vi "Save Analyzed Booth.vi"(8 "Error In":errorcluster, 10 "File Path":path, 11 "Data cluster":T1) -> (0 "Error Out":errorcluster)   [LabVIEW 2019, in "SubVIs.lvlib"]
uses:
  SubVIs.lvlib
  Controls/Save Data Cluster.ctl
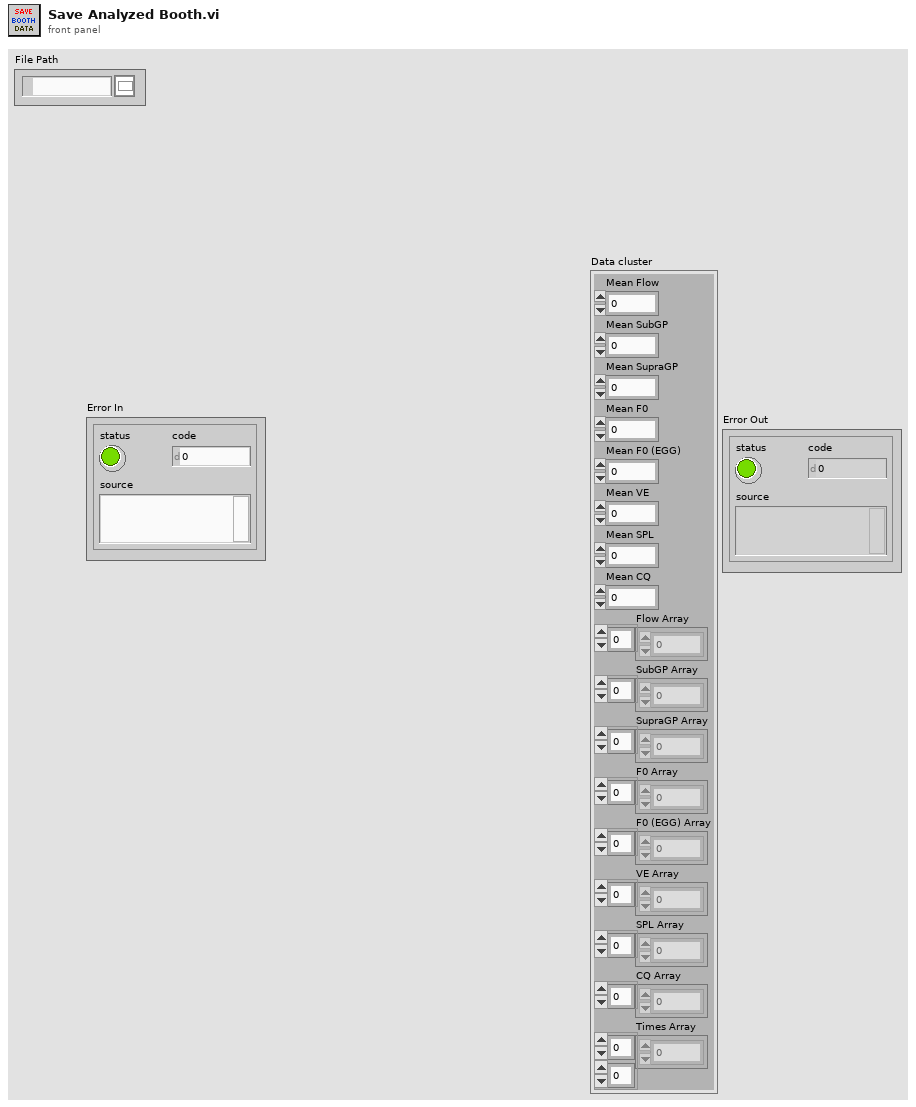
[diagram p1: front panel]
types:
  T1 = typedef "Save Data Cluster.ctl" = cluster{"Mean Flow":dbl, "Mean SubGP":dbl, "Mean SupraGP":dbl, "Mean F0":dbl, "Mean F0 (EGG)":dbl, "Mean VE":dbl, "Mean SPL":dbl, "Mean CQ":dbl, "Flow Array":dbl[], "SubGP Array":dbl[], "SupraGP Array":dbl[], "F0 Array":dbl[], "F0 (EGG) Array":dbl[], "VE Array":dbl[], "SPL Array":dbl[], "CQ Array":dbl[], "Times Array":dbl[][]}
  T2 = enum16{"open", "replace", "create", "open or create", "replace or create", "replace or create with confirmation"}
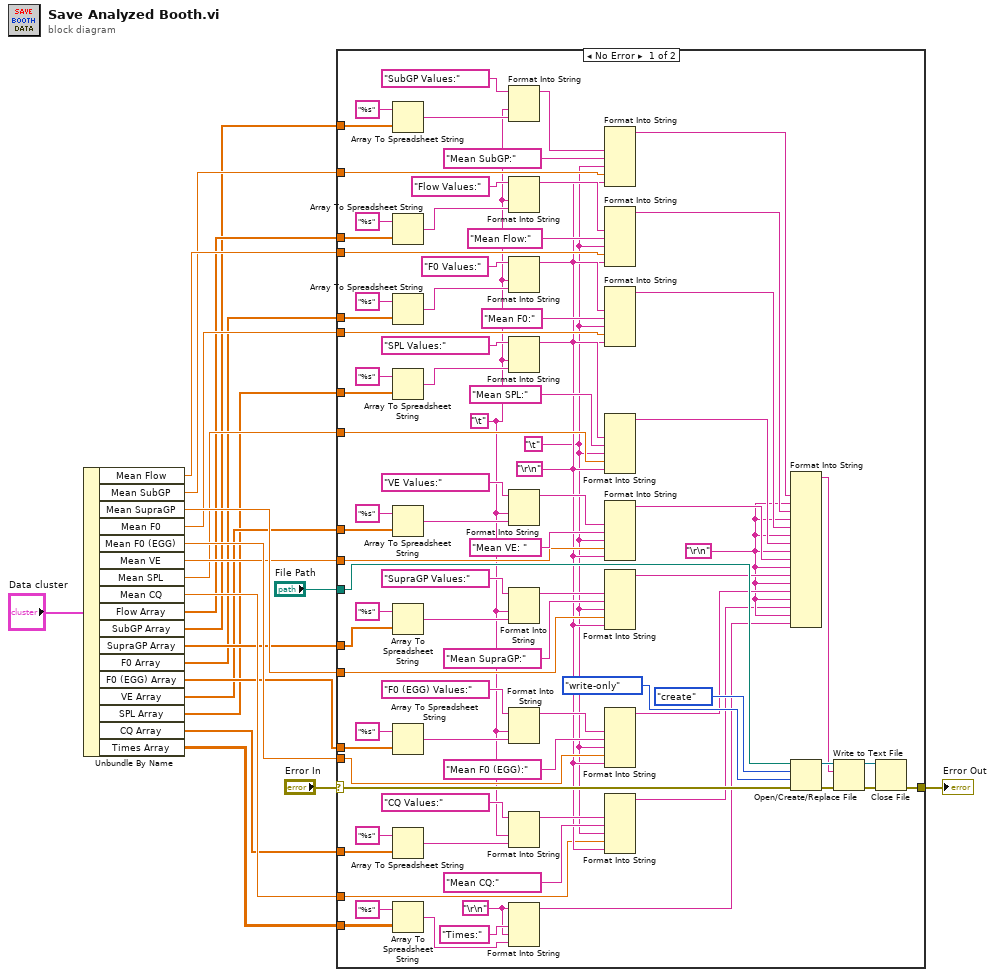
[diagram p0: block diagram]
diagram:
  n1 = Unbundle By Name("Data cluster") -> ("Mean Flow"=w16:dbl, "Mean SubGP"=w15:dbl, "Mean SupraGP"=w14:dbl, "Mean F0"=w13:dbl, "Mean F0 (EGG)"=w12:dbl, "Mean VE"=w11:dbl, "Mean SPL"=w10:dbl, "Mean CQ"=w9:dbl, "Flow Array"=w7:dbl[], "SubGP Array"=w6:dbl[], "SupraGP Array"=w5:dbl[], "F0 Array"=w4:dbl[], "F0 (EGG) Array"=w3:dbl[], "VE Array"=w2:dbl[], "SPL Array"=w1:dbl[], "CQ Array"=w8:dbl[], "Times Array"=w17:dbl[][])
  n2 = case shown="No Error" "Error In" {
    selector: "Error In" -> [w100 w106]
    tunnel: [w99 w106] -> w20
    tunnel: "File Path" -> [w105 _]
    tunnel: w17 -> [w49 _]
    tunnel: w16 -> [w48 _]
    tunnel: w15 -> [w47 _]
    tunnel: w14 -> [w46 _]
    tunnel: w13 -> [w45 _]
    tunnel: w12 -> [w44 _]
    tunnel: w11 -> [w43 _]
    tunnel: w10 -> [w42 _]
    tunnel: w9 -> [w32 _]
    tunnel: w8 -> [w30 _]
    tunnel: w7 -> [w28 _]
    tunnel: w6 -> [w27 _]
    tunnel: w5 -> [w26 _]
    tunnel: w4 -> [w25 _]
    tunnel: w3 -> [w24 _]
    tunnel: w2 -> [w23 _]
    tunnel: w1 -> [w22 _]
    frame No Error {
      w62 = "\r\n"
      w41 = "\r\n"
      w33 = "\t"
      w31 = "\t"
      w34 = "\r\n"
      n3 = Array To Spreadsheet String(array=w27, 3:"%s" ("format string")) -> (spreadsheet string=w86:string)  [unwired: 1 in]
      n4 = Array To Spreadsheet String(array=w28, 3:"%s" ("format string")) -> (spreadsheet string=w82:string)  [unwired: 1 in]
      n5 = Array To Spreadsheet String(array=w25, 3:"%s" ("format string")) -> (spreadsheet string=w83:string)  [unwired: 1 in]
      n6 = Array To Spreadsheet String(array=w22, 3:"%s" ("format string")) -> (spreadsheet string=w85:string)  [unwired: 1 in]
      n7 = Array To Spreadsheet String(array=w23, 3:"%s" ("format string")) -> (spreadsheet string=w84:string)  [unwired: 1 in]
      n8 = Array To Spreadsheet String(array=w26, 3:"%s" ("format string")) -> (spreadsheet string=w59:string)  [unwired: 1 in]
      n9 = Array To Spreadsheet String(array=w24, 3:"%s" ("format string")) -> (spreadsheet string=w53:string)  [unwired: 1 in]
      n10 = Array To Spreadsheet String(array=w30, 3:"%s" ("format string")) -> (spreadsheet string=w37:string)  [unwired: 1 in]
      n11 = Array To Spreadsheet String(array=w49, 3:"%s" ("format string")) -> (spreadsheet string=w64:string)  [unwired: 1 in]
      n12 = Format Into String(initial string="SubGP Values:", w31, w86) -> (resulting string=w81:string)  [unwired: 2 in, 1 out]
      n13 = Format Into String(initial string="Flow Values:", w31, w82) -> (resulting string=w80:string)  [unwired: 2 in, 1 out]
      n14 = Format Into String(initial string="F0 Values:", w31, w83) -> (resulting string=w79:string)  [unwired: 2 in, 1 out]
      n15 = Format Into String(initial string="SPL Values:", w31, w85) -> (resulting string=w78:string)  [unwired: 2 in, 1 out]
      n16 = Format Into String(initial string="VE Values:", w31, w84) -> (resulting string=w77:string)  [unwired: 2 in, 1 out]
      n17 = Format Into String(initial string="SupraGP Values:", w31, w59) -> (resulting string=w58:string)  [unwired: 2 in, 1 out]
      n18 = Format Into String(initial string="F0 (EGG) Values:", w31, w53) -> (resulting string=w52:string)  [unwired: 2 in, 1 out]
      n19 = Format Into String(initial string="CQ Values:", w31, w37) -> (resulting string=w36:string)  [unwired: 2 in, 1 out]
      n20 = Format Into String(initial string=w62, "Times:", w62, w64) -> (resulting string=w40:string)  [unwired: 2 in, 1 out]
      n21 = Format Into String(w81, "Mean SubGP:", w33, w47, w34) -> (resulting string=w76:string)  [unwired: 3 in, 1 out]
      n22 = Format Into String(w80, "Mean Flow:", w33, w48, w34) -> (resulting string=w75:string)  [unwired: 3 in, 1 out]
      n23 = Format Into String(w79, "Mean F0:", w33, w45, w34) -> (resulting string=w74:string)  [unwired: 3 in, 1 out]
      n24 = Format Into String(w78, "Mean SPL:", w33, w42, w34) -> (resulting string=w73:string)  [unwired: 3 in, 1 out]
      n25 = Format Into String(w77, "Mean VE: ", w33, w43, w34) -> (resulting string=w72:string)  [unwired: 3 in, 1 out]
      n26 = Format Into String(w58, "Mean SupraGP:", w33, w46, w34) -> (resulting string=w56:string)  [unwired: 3 in, 1 out]
      n27 = Format Into String(w52, "Mean F0 (EGG):", w33, w44, w34) -> (resulting string=w50:string)  [unwired: 3 in, 1 out]
      n28 = Format Into String(w36, "Mean CQ:", w33, w32, w34) -> (resulting string=w29:string)  [unwired: 3 in, 1 out]
      n29 = Format Into String(w76, w41, w75, w41, w74, w41, w73, w41, w72, w41, w56, w41, w50, w41, w29, w41, w40) -> (resulting string=w71:string)  [unwired: 3 in, 1 out]
      n30 = Open/Create/Replace File(file path (use dialog)=w105, error in=w100, operation (0:open)=T2."create", access (0:read/write)=enum16{"read/write", "read-only", "write-only"}."write-only") -> (refnum out=w102:refnum<file>, error out=w101:errorcluster)  [unwired: 2 in, 1 out]
      n31 = Write to Text File(file (use dialog)=w102, text=w71, error in=w101) -> (refnum out=w98:refnum<file>, error out=w97:errorcluster)  [unwired: 1 in, 1 out]
      n32 = Close File(refnum=w98, error in=w97) -> (error out=w99:errorcluster)  [unwired: 1 out]
    }
    frame Error {
    }
  }
  "Error Out" <- w20
